vi "Arduino Debug Program.vi"() -> ()   [LabVIEW 2024, in "FW Arduino Control.lvclass"]
uses:
  FW Arduino Control.lvclass
  Debug Program Settings.ctl
  Filter Wheel Arduino Homing cluster.ctl
panel:
  in  "Homing Parameters":T1
  out "after substring 2":string
  out "after substring":string
  out "number":i32
  out "response":string
  in  "Homing Parameters old":T2={"Direction (F: CW)"=TRUE, "Speed"=150, "Accel"=400, "Error Cnts"=100, "Homing Deltas"=[3000, 3000, -680, -1560]}
  out "Move Distance":i32
  out "Moving":bool
  in  "Clear History":bool
  in  "Defaults":T3={"VISA resource name"="COM9", "Speed"=400, "Ramp Slope"=400, "Motor ID (0:n-1)"=0, "baud rate"=9600}
  in  "Close":bool
  out "Arduino Responses":string
  out "Last Command":string
  in  "Command":string
  in  "Send":bool
  in  "Home Button":bool
  in  "Move":bool
  in  "Counts to Move":i32=1400
  # "Commanding"
  # "Home speed max 200\nor the indentations\nmay be missed."
  # "*  Check communications:\n *      [C]|[check code]|[EOT]\n *\n *  Move:\n *      [M]|Motor # [0-3]|Motor State [1]|Motor Direction [+,-]|Type of Move [R,S]|# Steps [uint]|Delimiter [:]|Max. Rate [uint]|Delimiter [:]|Ramp Slope [uint]|Delimiter [:] (optional)|# Positions [uint] (optional)|[EOT]\n *          * type of move: R --> relative move, S --> switch move\n *          * if number of steps is 0 --> free run\n *          * if Ramp Slope == 0 -> no ramp (start at max. rate)\n *          * may specify the number of position to move for a switch move.  if not specified, defaults to 1 position.\n *\n *  Emergency Stop:\n *      [M]|Motor # [0-3]|Motor State [0]|[EOT]\n *\n *  Get Motor Completed Steps:\n *      [Q]|Motor # [0-3]|[C]|[EOT]\n *  Get Motor Direction:\n *      [Q]|Motor # [0-3]|[D]|[EOT]\n *  Get Motor Step Rate:\n *      [Q]|Motor # [0-3]|[R]|[EOT]\n *  Get Switch State:\n *      [Q]|Motor # [0-3]|[S]|[EOT]\n *\n *  Set Emergency Ramp Multiplier:\n *      [V]|Motor # [0-3]|[E]|Multiplier [uint]|[EOT]\n */"
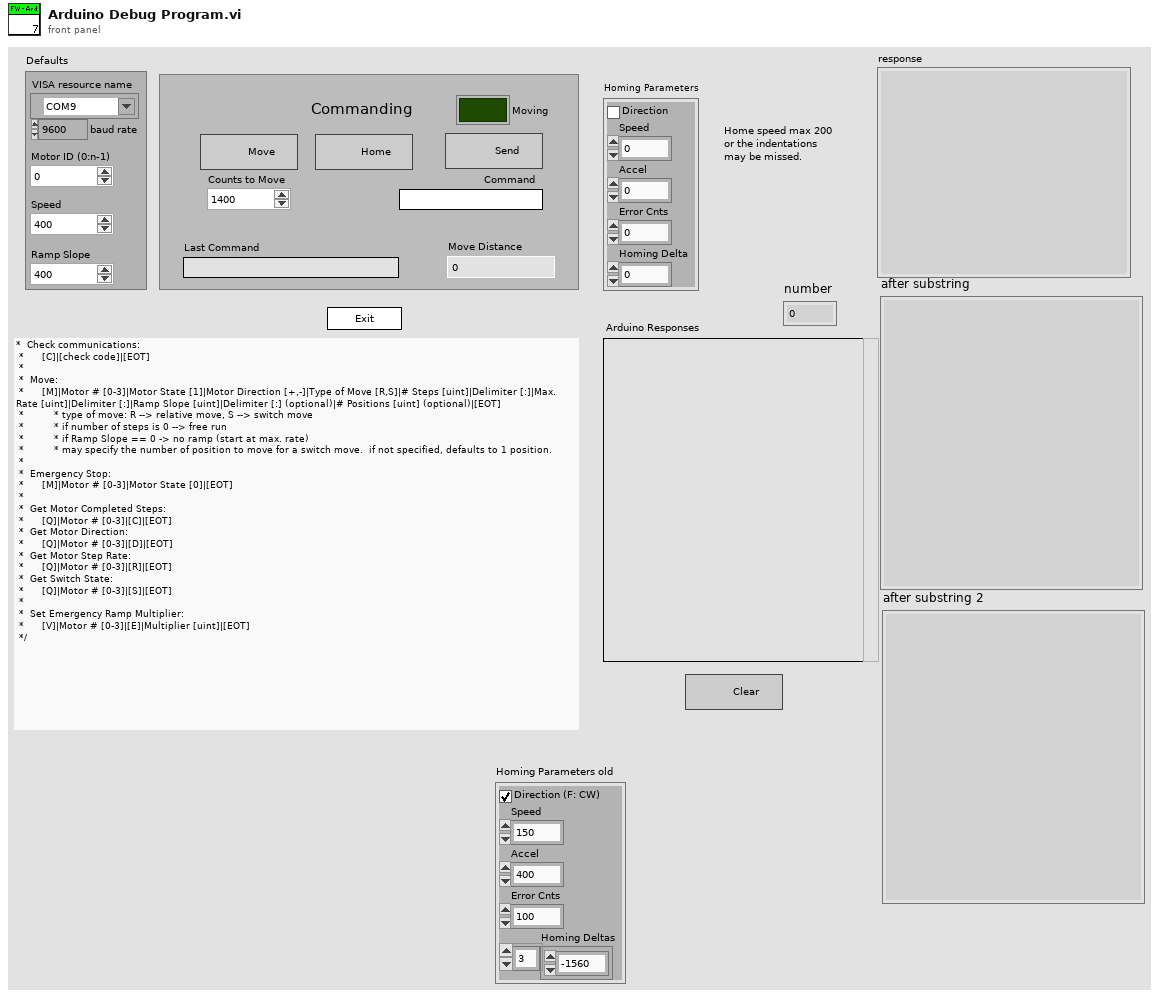
[diagram p1: front panel]
types:
  T1 = typedef "Filter Wheel Arduino Homing cluster.ctl" = cluster{"Direction":bool, "Speed":i32, "Accel":i32, "Error Cnts":i32, "Homing Delta":i32}
  T2 = cluster{"Direction (F: CW)":bool, "Speed":i32, "Accel":i32, "Error Cnts":i32, "Homing Deltas":i32[]}
  T3 = typedef "Debug Program Settings.ctl" = cluster{"VISA resource name":refnum<visa-resource-name>, "Speed":i32, "Ramp Slope":i32, "Motor ID (0:n-1)":i32, "baud rate":u32}
  T4 = cluster{"state":refnum<user-event>, "Defaults":T3, "cmd string":string, "connected":bool, "Moving":bool, "log ref":refnum<file>}
  T5 = enum32{"invalid app kind", "Development System", "Run Time System", "Student Edition", "Embedded LabVIEW", "Evaluation", "Custom"}
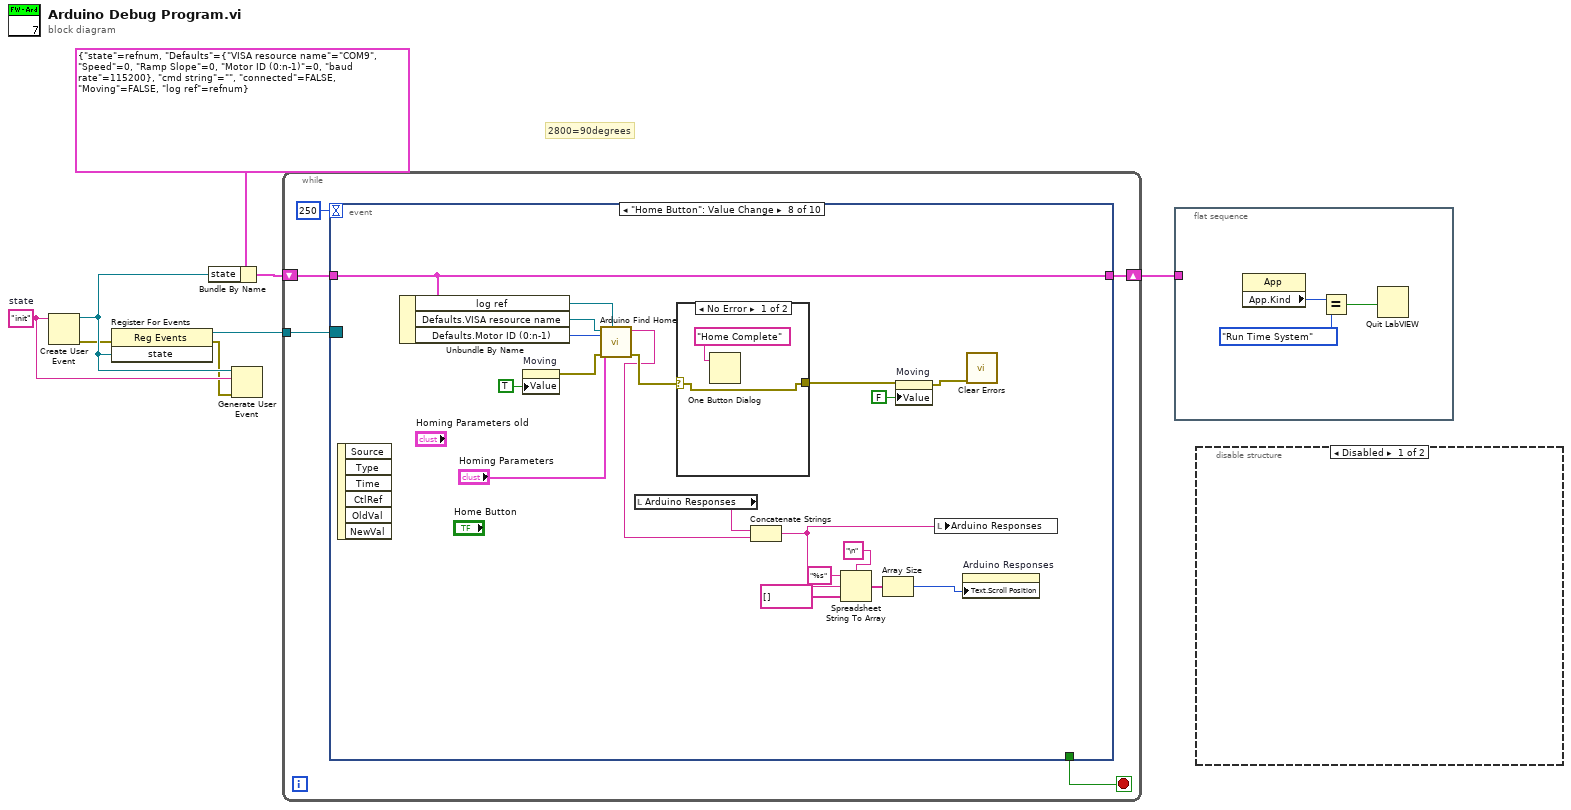
[diagram p0: block diagram]
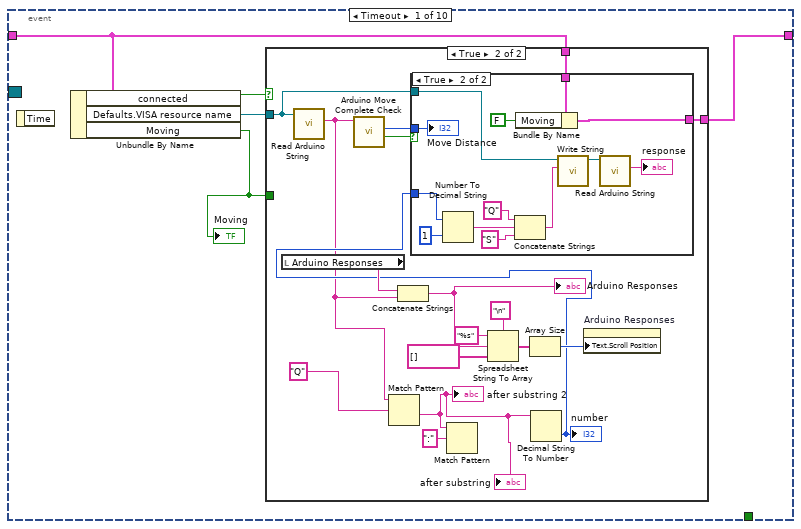
[diagram p3: hidden frame]
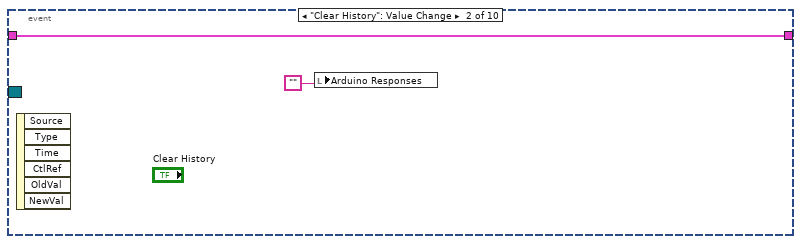
[diagram p6: hidden frame]
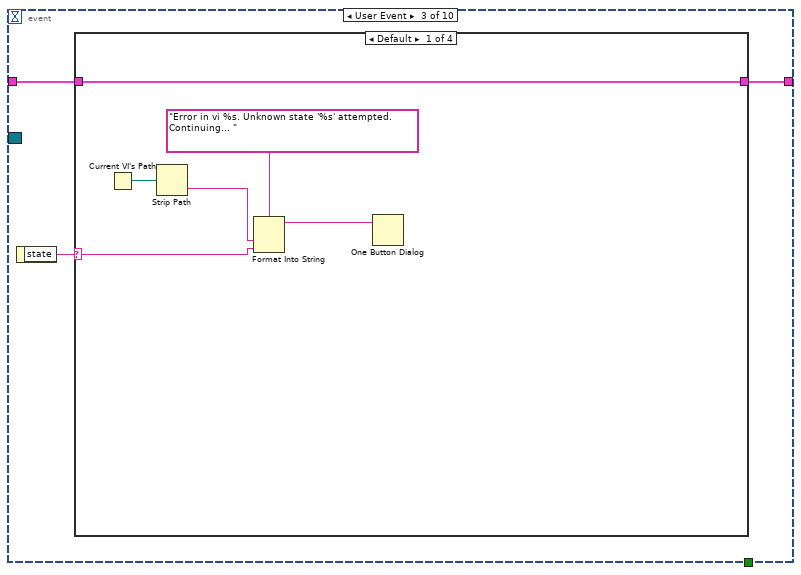
[diagram p7: hidden frame]
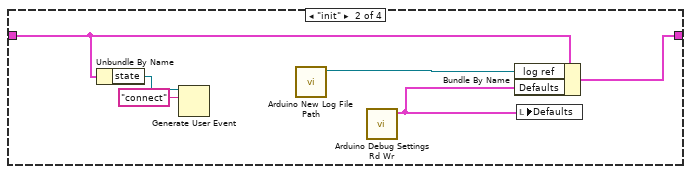
[diagram p8: hidden frame]
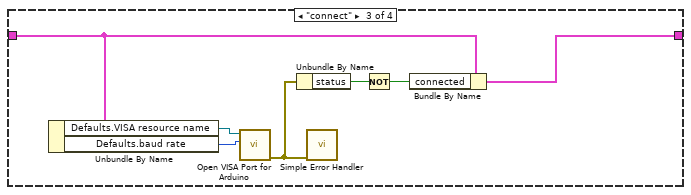
[diagram p9: hidden frame]
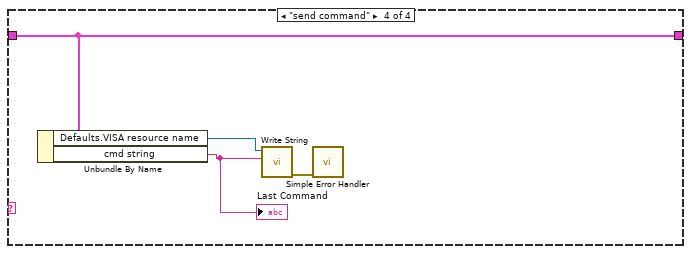
[diagram p10: hidden frame]
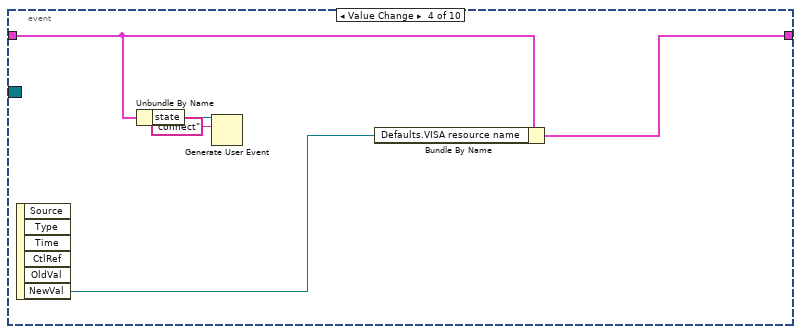
[diagram p11: hidden frame]
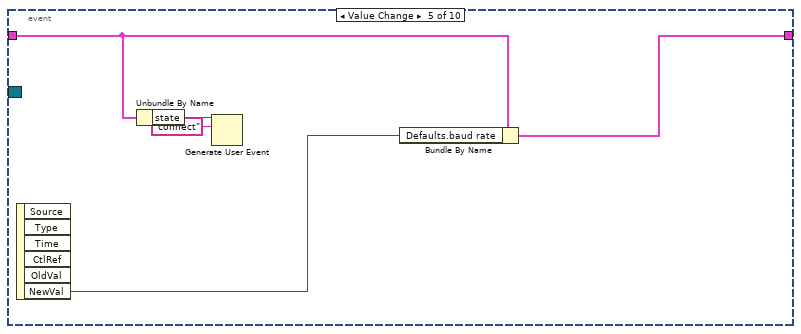
[diagram p12: hidden frame]
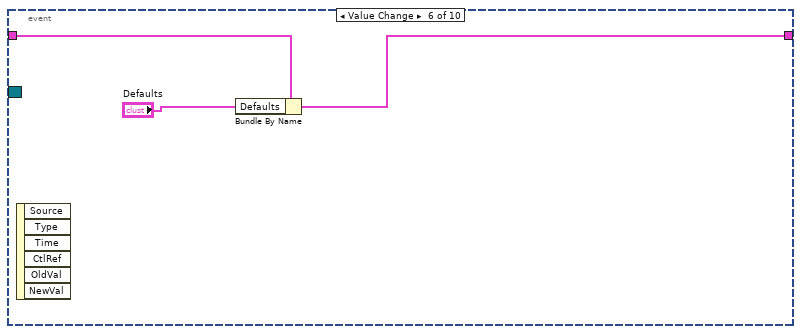
[diagram p13: hidden frame]
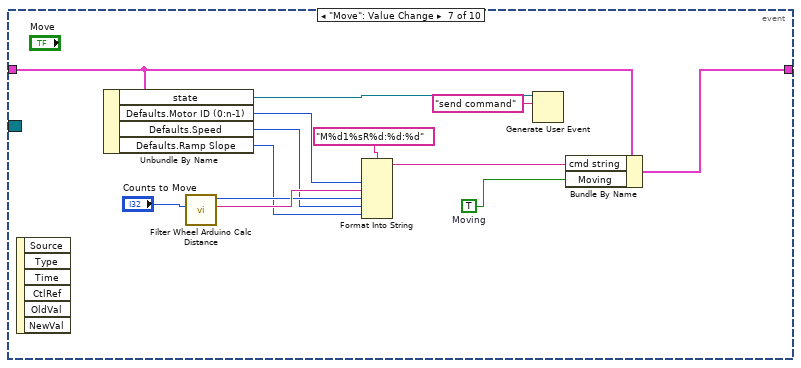
[diagram p14: hidden frame]
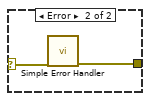
[diagram p15: hidden frame]
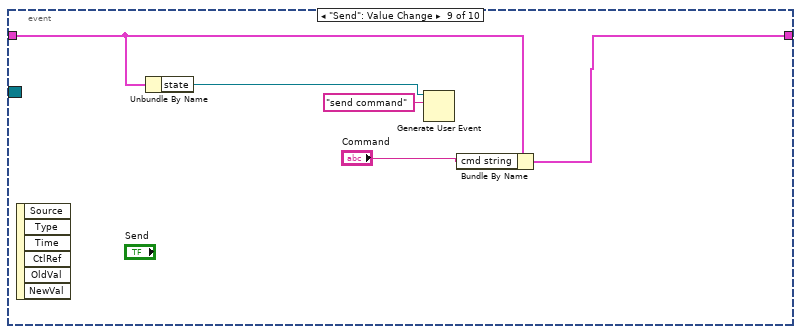
[diagram p16: hidden frame]
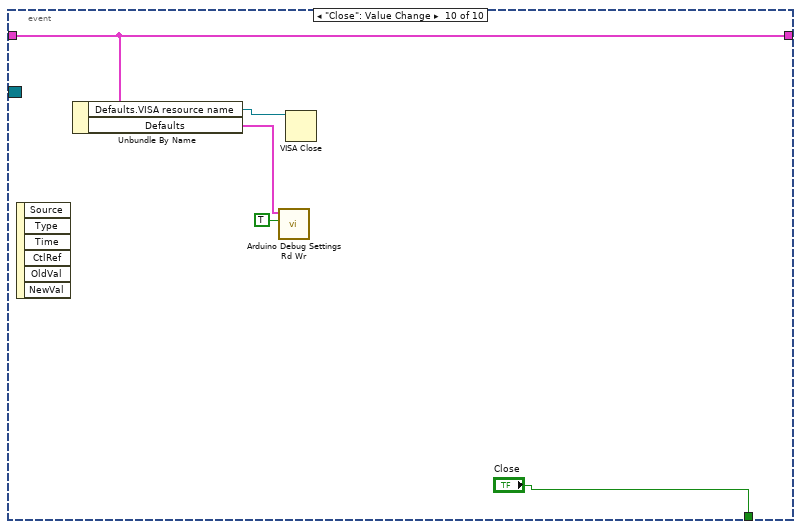
[diagram p17: hidden frame]
diagram:
  w4 = "init"  # state
  # "2800=90degrees"
  n1 = Create User Event(user event datatype=w4) -> (user event=w6:refnum<user-event>, error out=w2:errorcluster)  [unwired: 1 in]
  n2 = register-events(error in=w2, w6) -> (reference out=w5:refnum<event-registration>, error out=w3:errorcluster)  [unwired: 1 in]
  n3 = Bundle By Name(cluster=T4 {"state"=refnum, "Defaults"={"VISA resource name"="COM9", "Speed"=0, "Ramp Slope"=0, "Motor ID (0:n-1)"=0, "baud rate"=115200}, "cmd string"="", "connected"=FALSE, "Moving"=FALSE, "log ref"=refnum}, "state"=w6) -> (w7:T4)
  n4 = Generate User Event(user event=w6, event data cluster=w4, error in=w3) -> ()  [unwired: 1 in, 2 out]
  n5 = while {
    tunnel: w5 -> [w13]
    shift-right: [w11] -> w1
    shift-left: w7 -> [w12]
    stop <- w10 stop-if-true
    n6 = event shown="[7] \"Home Button\": Value Change" {
      selector: w13 -> [_ _ _ _ _ _ _ _ _ _]
      dyn-events: _ -> [_ _ _ _ _ _ _ _ _ _]
      timeout: 250 -> [_ _ _ _ _ _ _ _ _ _]
      tunnel: w12 -> [w15 w52 w54 w79 w84 w89 w97 w119 w130 w136]
      tunnel: [w16 w52 w53 w80 w85 w90 w93 w119 w131 w136] -> w11
      tunnel: [_ _ _ _ _ _ _ _ _ "Close"] -> w10
      event Timeout {
        n7 = event-data() -> ()  [unwired: 1 in, 1 out]
        n8 = Unbundle By Name(w15) -> ("connected"=w18:bool, "Defaults.VISA resource name"=w17:refnum<visa-resource-name>, "Moving"=w14:bool)
        "Moving" <- w14
        n9 = case shown="True" w18 {
          tunnel: w17 -> [_ w23]
          tunnel: w14 -> [_ _]
          tunnel: w15 -> [w19 w29]
          tunnel: [w19 w27] -> w16
          frame False {
          }
          frame True {
            n10 = local read "Arduino Responses"() -> (w36:string)
            n11 = call "Read Arduino String.vi"("reference"=w23) -> ("response"=w20:string)  [unwired: 8 in, 2 out]
            n12 = call "Arduino Move Complete Check.vi"("input string"=w20) -> ("Complete?"=w30:bool, "position"=w28:i32)  [unwired: 7 in, 2 out]
            n13 = Match Pattern(string=w20, regular expression="Q") -> (after substring=w22:string)  [unwired: 1 in, 3 out]
            "after substring" <- w22
            "after substring 2" <- w22
            n14 = Concatenate Strings(w36, w20) -> (w26:string)
            "Arduino Responses" <- w26
            n15 = Match Pattern(string=w22, regular expression=":") -> ()  [unwired: 1 in, 4 out]
            n16 = Spreadsheet String To Array(delimiter (Tab)="\n", format string="%s", spreadsheet string=w26, array type (2D Dbl)=string[] []) -> (array=w33:string[])
            n17 = Array Size(array=w33) -> (size(s)=w31:i32)
            n18 = Decimal String To Number(string=w22) -> (number=w21:i32)  [unwired: 2 in, 1 out]
            "number" <- w21
            n19 = case shown="True" w30 {
              tunnel: w29 -> [w37 w50]
              tunnel: w28 -> [_ w47]
              tunnel: [w37 w48] -> w27
              tunnel: w23 -> [_ w39]
              tunnel: w21 -> [_ w38]
              frame False {
              }
              frame True {
                n20 = Number To Decimal String(number=w38, width (-)=i16 1) -> (decimal integer string=w46:string)
                n21 = Concatenate Strings("Q", w46, "S") -> (w43:string)
                n22 = Bundle By Name(cluster=w50, "Moving"=FALSE) -> (w48:T4)
                n23 = call "Write String.vi"("String"=w43, "VISA resource name"=w39) -> ("VISA resource name out"=w44:refnum<visa-resource-name>)  [unwired: 8 in, 1 out]
                n24 = call "Read Arduino String.vi"("reference"=w44) -> ("response"=→"response":string)  [unwired: 8 in, 2 out]
                "Move Distance" <- w47
              }
            }
            n25 = property on="Arduino Responses" class="Str"("Text.Scroll Position"=w31) -> ()  [unwired: 2 in, 2 out]
          }
        }
      }
      event "Clear History": Value Change {
        n26 = event-data() -> ()  [unwired: 1 in, 6 out]
        n27 = local write "Arduino Responses"("") -> ()
      }
      event User Event {
        n28 = event-data() -> ("state"=w55:string)  [unwired: 1 in]
        n29 = case shown="Default" w55 {
          selector: w55 -> [w60 _ _ _]
          tunnel: w54 -> [w56 w65 w69 w78]
          tunnel: [w56 w66 w70 w78] -> w53
          frame Default {
            n30 = Current VI's Path() -> (path=w59:path)
            n31 = Strip Path(path=w59) -> (name=w58:string)  [unwired: 1 out]
            n32 = Format Into String(format string="Error in vi %s. Unknown state '%s' attempted. Continuing... ", w58, w60) -> (resulting string=w57:string)  [unwired: 2 in, 1 out]
            n33 = One Button Dialog(message=w57) -> ()  [unwired: 1 in, 1 out]
          }
          frame "init" {
            n34 = Unbundle By Name(w65) -> ("state"=w64:refnum<user-event>)
            n35 = Generate User Event(user event=w64, event data cluster="connect" ("event data")) -> ()  [unwired: 2 in, 2 out]
            n36 = call "Arduino New Log File Path.vi"() -> ("log ref"=w62:refnum<file>)  [unwired: 11 in]
            n37 = call "Arduino Debug Settings Rd Wr.vi"() -> ("Defaults"=w67:T3)  [unwired: 10 in, 1 out]
            n38 = Bundle By Name(cluster=w65, "log ref"=w62, "Defaults"=w67) -> (w66:T4)
            n39 = local write "Defaults"(w67) -> ()
          }
          frame "connect" {
            n40 = Unbundle By Name(w69) -> ("Defaults.VISA resource name"=w74:refnum<visa-resource-name>, "Defaults.baud rate"=w68:u32)
            n41 = call "Open VISA Port for Arduino.vi"("baud rate (9600)"=w68, "VISA resource name"=w74) -> ("error out"=w73:errorcluster)  [unwired: 8 in, 1 out]
            n42 = Unbundle By Name(w73) -> ("status"=w72:bool)
            n43 = call <vilib>:"Simple Error Handler.vi"("error in (no error)"=w73) -> ()  [unwired: 4 in, 5 out]
            n44 = Not(x=w72) -> (.not. x?=w71:bool)
            n45 = Bundle By Name(cluster=w69, "connected"=w71) -> (w70:T4)
          }
          frame "send command" {
            n46 = Unbundle By Name(w78) -> ("Defaults.VISA resource name"=w77:refnum<visa-resource-name>, "cmd string"=w76:string)
            "Last Command" <- w76
            n47 = call "Write String.vi"("String"=w76, "VISA resource name"=w77) -> ("error out"=w75:errorcluster)  [unwired: 8 in, 1 out]
            n48 = call <vilib>:"Simple Error Handler.vi"("error in (no error)"=w75) -> ()  [unwired: 4 in, 5 out]
          }
        }
      }
      event Value Change {
        n49 = event-data() -> ("NewVal"=w81:refnum<visa-resource-name>)  [unwired: 1 in, 5 out]
        n50 = Unbundle By Name(w79) -> ("state"=w83:refnum<user-event>)
        n51 = Generate User Event(user event=w83, event data cluster="connect" ("event data")) -> ()  [unwired: 2 in, 2 out]
        n52 = Bundle By Name(cluster=w79, "Defaults.VISA resource name"=w81) -> (w80:T4)
      }
      event Value Change {
        n53 = event-data() -> ("NewVal"=w86:u32)  [unwired: 1 in, 5 out]
        n54 = Unbundle By Name(w84) -> ("state"=w88:refnum<user-event>)
        n55 = Generate User Event(user event=w88, event data cluster="connect" ("event data")) -> ()  [unwired: 2 in, 2 out]
        n56 = Bundle By Name(cluster=w84, "Defaults.baud rate"=w86) -> (w85:T4)
      }
      event Value Change {
        n57 = event-data() -> ()  [unwired: 1 in, 6 out]
        n58 = Bundle By Name(cluster=w89, "Defaults"="Defaults") -> (w90:T4)
      }
      event "Move": Value Change {
        w94 = TRUE  # Moving
        n59 = event-data() -> ()  [unwired: 1 in, 6 out]
        n60 = Unbundle By Name(w97) -> ("state"=w96:refnum<user-event>, "Defaults.Motor ID (0:n-1)"=w92:i32, "Defaults.Speed"=w100:i32, "Defaults.Ramp Slope"=w99:i32)
        n61 = call "Filter Wheel Arduino Calc Distance.vi"("To Position"="Counts to Move") -> ("Direction"=w102:string, "Counts"=w101:u32)  [unwired: 8 in, 1 out]
        n62 = Format Into String(format string="M%d1%sR%d:%d:%d", w92, w102, w101, w100, w99) -> (resulting string=w98:string)  [unwired: 2 in, 1 out]
        n63 = Generate User Event(user event=w96, event data cluster="send command" ("event data")) -> ()  [unwired: 2 in, 2 out]
        n64 = Bundle By Name(cluster=w97, "cmd string"=w98, "Moving"=w94) -> (w93:T4)
      }
      event "Home Button": Value Change {
        n65 = event-data() -> ()  [unwired: 1 in, 6 out]
        n66 = Unbundle By Name(w119) -> ("log ref"=w106:refnum<file>, "Defaults.VISA resource name"=w123:refnum<visa-resource-name>, "Defaults.Motor ID (0:n-1)"=w122:i32)
        n67 = property on="Moving" class="Bool (strict)"("Value"=TRUE ("Moving")) -> (error out=w121:errorcluster)  [unwired: 2 in, 1 out]
        n68 = call "Arduino Find Home.vi"("log ref"=w106, "error in"=w121, "Homing Parameters"="Homing Parameters", "Motor"=w122, "Addr"=w123) -> ("error out"=w118:errorcluster, "Log"=w110:string)  [unwired: 4 in, 1 out]
        n69 = local read "Arduino Responses"() -> (w115:string)
        n70 = case shown="No Error" w118 {
          selector: w118 -> [w124 w127]
          tunnel: [w124 w126] -> w117
          frame No Error {
            n71 = One Button Dialog(message="Home Complete") -> ()  [unwired: 1 in, 1 out]
          }
          frame Error {
            n72 = call <vilib>:"Simple Error Handler.vi"("error in (no error)"=w127) -> ("error out"=w126:errorcluster)  [unwired: 4 in, 4 out]
          }
        }
        n73 = Concatenate Strings(w115, w110) -> (w109:string)
        n74 = Spreadsheet String To Array(delimiter (Tab)="\n", format string="%s", spreadsheet string=w109, array type (2D Dbl)=string[] []) -> (array=w114:string[])
        n75 = Array Size(array=w114) -> (size(s)=w108:i32)
        n76 = property on="Moving" class="Bool (strict)"(error in=w117, "Value"=FALSE ("Moving")) -> (error out=w107:errorcluster)  [unwired: 1 in, 1 out]
        n77 = local write "Arduino Responses"(w109) -> ()
        n78 = property on="Arduino Responses" class="Str"("Text.Scroll Position"=w108) -> ()  [unwired: 2 in, 2 out]
        n79 = call <vilib>:"Clear Errors.vi"("error in (no error)"=w107) -> ()  [unwired: 5 in, 2 out]
      }
      event "Send": Value Change {
        n80 = event-data() -> ()  [unwired: 1 in, 6 out]
        n81 = Unbundle By Name(w130) -> ("state"=w129:refnum<user-event>)
        n82 = Generate User Event(user event=w129, event data cluster="send command" ("event data")) -> ()  [unwired: 2 in, 2 out]
        n83 = Bundle By Name(cluster=w130, "cmd string"="Command") -> (w131:T4)
      }
      event "Close": Value Change {
        n84 = event-data() -> ()  [unwired: 1 in, 6 out]
        n85 = Unbundle By Name(w136) -> ("Defaults.VISA resource name"=w135:refnum<visa-resource-name>, "Defaults"=w134:T3)
        n86 = call "Arduino Debug Settings Rd Wr.vi"("Write? (F:Read)"=TRUE, "Defaults"=w134) -> ()  [unwired: 8 in, 2 out]
        n87 = VISA Close(VISA resource name=w135) -> ()  [unwired: 1 in, 1 out]
      }
    }
  }
  n88 = flat-sequence {
    tunnel: w1 -> [_]
    frame #0 {
      n89 = property class="App"() -> ("App.Kind"=w140:T5)  [unwired: 2 in, 2 out]
      n90 = Equal?(x=w140, y=T5."Run Time System") -> (x = y?=w138:bool)
      n91 = Quit LabVIEW(quit? (T)=w138) -> ()
    }
  }
  n92 = disable-structure shown="Disabled" {
    frame Disabled {
    }
    frame Enabled {
    }
  }
